vi "Reload Config.vi"(8 "error in (no error)":errorcluster, 9 "Promise":refnum<class "Promise.lvclass">, 10 "Config Type":string, 11 "DaqControl in":refnum<class "DaqControl.lvclass">) -> (0 "error out":errorcluster, 3 "DaqControl out":refnum<class "DaqControl.lvclass">)   [LabVIEW 2020, in "VolatusDaq.lvlib" / "DaqControl.lvclass"]
uses:
  DaqControl.lvclass
  lv-promises/Promises/Promise/Promise.lvclass
  DaqControl.lvclass/DaqControl.ctl
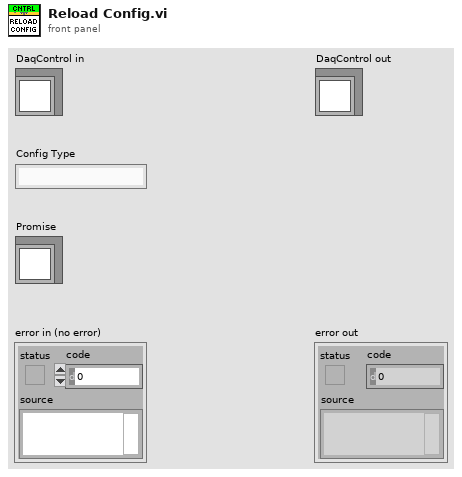
[diagram p1: front panel]
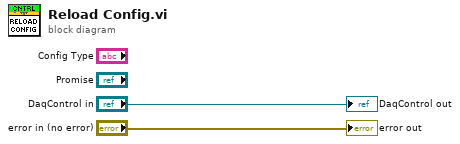
[diagram p0: block diagram]
diagram:
  "error out" <- "error in (no error)"
  "DaqControl out" <- "DaqControl in"
